vi "Engine-Channels.vi"(8 "error in (no error)":errorcluster, 11 "DSI Reference":refnum<class "DCM-DSI.lvclass">) -> (0 "error out":errorcluster, 3 "DSI Reference":refnum<class "DCM-DSI.lvclass">)   [LabVIEW 2016, in "DSI-RT.lvlib"]
uses:
  DSI-RT.lvlib
  Classes/DCM-DSI/DCM-DSI.lvclass
  Classes/DCM-DSI/Read Channels.vi
  <vilib>/addons/Software Calibration Management/xSCM/CalPoint.xnode
  <vilib>/addons/Software Calibration Management/xSCM/ni_scm.dll
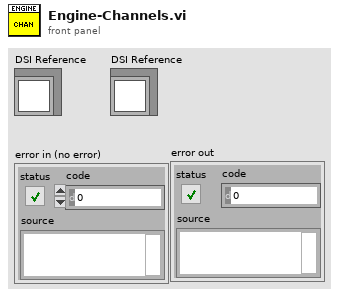
[diagram p1: front panel]
types:
  T1 = typedef "DCM-DSI.lvclass/Channel.ctl" = cluster{"Name":string, "Unit":string, "Value":sgl}
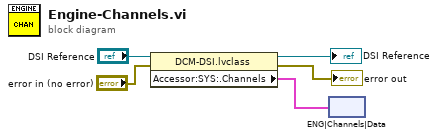
[diagram p0: block diagram]
diagram:
  n1 = property class="DCM-DSI.lvclass"(reference="DSI Reference", error in="error in (no error)") -> (reference out=→"DSI Reference":refnum<class "DCM-DSI.lvclass">, error out=→"error out":errorcluster, "Accessor:SYS:.Channels"=w2:T1[])
  n2 = xnode "ENG|Channels|Data"("Value"=w2) -> ()
